vi "Hitrap_DiagnosticBox.get diagnosticparameters.vi"(0 "i ref in":refnum<vi>, 5 "error in (no error)":errorcluster) -> (14 "i ref out":refnum<vi>, 16 "appended array":string[](array[string]), 19 "error out":errorcluster)   [LabVIEW 2014, in "Hitrap_DiagnosticBox.lvlib"]
doc: "gets the diagnostic parameters required for the axis."
uses:
  Hitrap_DiagnosticBox.lvlib
  CS_Core/BaseProcess/BaseProcess.lvlib
  CS_Core/CSSystem/CoreLib/CoreLib.lvlib
  CS_Motion/NanotecSMCPD/NanotecSMCPD.lvlib
panel:
  in  "Diagnostic":T1
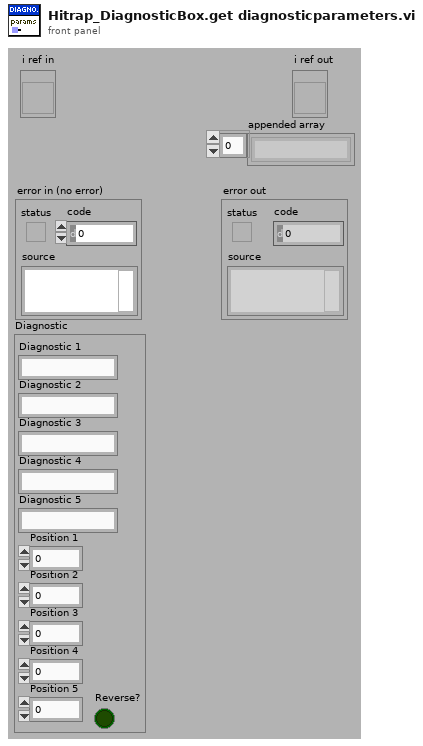
[diagram p1: front panel]
types:
  T1 = cluster{"Diagnostic 1":string, "Diagnostic 2":string, "Diagnostic 3":string, "Diagnostic 4":string, "Diagnostic 5":string, "Position 1":dbl, "Position 2":dbl, "Position 3":dbl, "Position 4":dbl, "Position 5":dbl, "Reverse?":bool}
  T2 = typedef "BaseProcess.lvlib/BaseProcess.i attribute.ctl" = cluster{"EventStatus":string, "EventError":i32, "PresetEvtWatchD":i32, "PresetPdcWatchD":i32, "EventTimeout":i32, "PeriodicInterval":i32, "Interface":string[], "Address":string[], "Special":string[], "PeriodicError":i32, "PeriodicStatus":string, "SuperProc":string, "Descriptors":T3[], "CaseRef":refnum<vi>, "PdcRef":refnum<vi>, "Thread Ref":refnum<vi>, "eventErrorID":i32, "eventStatusID":i32, "periodicErrorID":i32, "periodicStatusID":i32, "pdcCtrID":i32}
  T3 = typedef "BaseProcess.lvlib/BaseProcess.descriptor definition.ctl" = cluster{"selector":string, "descriptor":T4}
  T4 = typedef "BaseProcess.lvlib/BaseProcess.descriptor string definition.ctl" = string
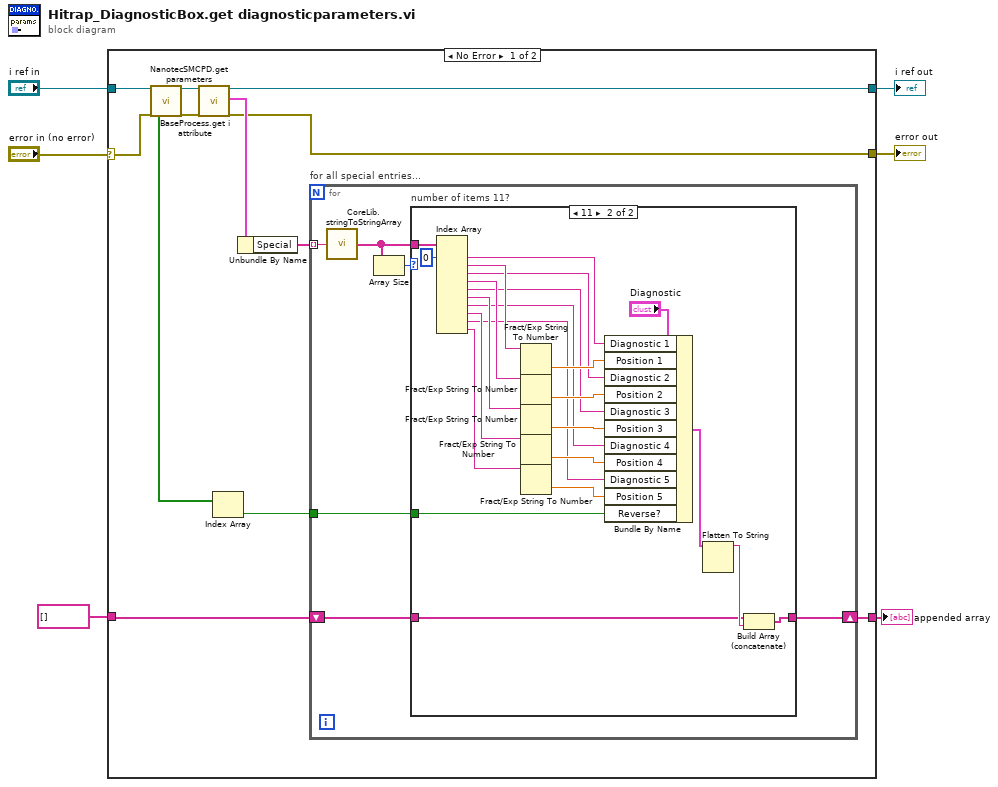
[diagram p0: block diagram]
diagram:
  n1 = case shown="No Error" "error in (no error)" {
    selector: "error in (no error)" -> [w10 w50]
    tunnel: "i ref in" -> [w9 w51]
    tunnel: [w17 w51] -> w5
    tunnel: [w16 w50] -> w4
    tunnel: [w14 w49] -> w1
    tunnel: string[] [] ("appended array") -> [w13 w49]
    frame No Error {
      n2 = call "NanotecSMCPD.get parameters.vi"("i ref in"=w9, "error in (no error)"=w10) -> ("ReverseDirection?"=w8:bool[], "i ref out"=w12:refnum<vi>, "error out"=w11:errorcluster)  [unwired: 6 in, 9 out]
      n3 = call "BaseProcess.get i attribute.vi"("i ref in"=w12, "error in (no error)"=w11) -> ("i ref out"=w17:refnum<vi>, "i attribute"=w18:T2, "error out"=w16:errorcluster)  [unwired: 15 in]
      n4 = Index Array(array=w8) -> (element=w7:bool)  [unwired: 1 in]
      n5 = Unbundle By Name(w18) -> ("Special"=w15:string[])
      n6 = for "for all special entries..." {
        tunnel: w15 -> [w24] mode=indexing
        shift-right: [w20] -> w14
        shift-left: w13 -> [w21]
        tunnel: w7 -> [w19]
        n7 = call "CoreLib.stringToStringArray.vi"("String"=w24) -> ("Array"=w22:string[])
        n8 = Array Size(array=w22) -> (size(s)=w23:i32)
        n9 = case "number of items 11?" shown="11" w23 {
          tunnel: w21 -> [w25 w28]
          tunnel: w22 -> [_ w48]
          tunnel: [w25 w27] -> w20
          tunnel: w19 -> [_ w26]
          frame 0, Default {
          }
          frame 11 {
            n10 = Index Array(array=w48, index #1=0 ("index")) -> (element #1=w45:string, element #2=w46:string, element #3=w31:string, element #4=w43:string, element #5=w32:string, element #6=w42:string, element #7=w33:string, element #8=w41:string, element #9=w34:string, element #10=w40:string)  [unwired: 9 in]
            n11 = Fract/Exp String To Number(string=w46) -> (number=w44:dbl)  [unwired: 3 in, 1 out]
            n12 = Fract/Exp String To Number(string=w43) -> (number=w38:dbl)  [unwired: 3 in, 1 out]
            n13 = Fract/Exp String To Number(string=w42) -> (number=w37:dbl)  [unwired: 3 in, 1 out]
            n14 = Fract/Exp String To Number(string=w41) -> (number=w36:dbl)  [unwired: 3 in, 1 out]
            n15 = Fract/Exp String To Number(string=w40) -> (number=w35:dbl)  [unwired: 3 in, 1 out]
            n16 = Bundle By Name(cluster="Diagnostic", "Diagnostic 1"=w45, "Position 1"=w44, "Diagnostic 2"=w31, "Position 2"=w38, "Diagnostic 3"=w32, "Position 3"=w37, "Diagnostic 4"=w33, "Position 4"=w36, "Diagnostic 5"=w34, "Position 5"=w35, "Reverse?"=w26) -> (w30:T1)
            n17 = Flatten To String(anything=w30) -> (data string=w29:string)  [unwired: 3 in, 2 out]
            n18 = Build Array (concatenate)(w28, w29) -> (w27:string[])
          }
        }
      }
    }
    frame Error {
    }
  }
  "error out" <- w4
  "i ref out" <- w5
  "appended array" <- w1
